vi "EditAxisSpaceCfg_Dialog.vi"(2 "error in":errorcluster, 3 "default save path":path) -> (0 "error out":errorcluster, 1 "Cancelled?":bool)   [LabVIEW 2009]
uses:
  typedefs/AxisSpaceCfg.ctl
  typedefs/AxisCfg.ctl
  globals/AxisSpace.vi
panel:
  in  "Export":bool
  in  "Import":bool
  in  "Cancel Button":bool
  in  "OK Button":bool
  in  "Axis Space":T1
  # "X-Axis\n(Axis 0)"
  # "Y-Axis\n(Axis 1)"
  # "Z-Axis\n(Axis 2)"
  # "Axis Space\n(Axis 3)"
  # "NOTE: \nThis is the \"broadcast axis\". The only value that is used here is the address which is used to broadcast commands to all axes."
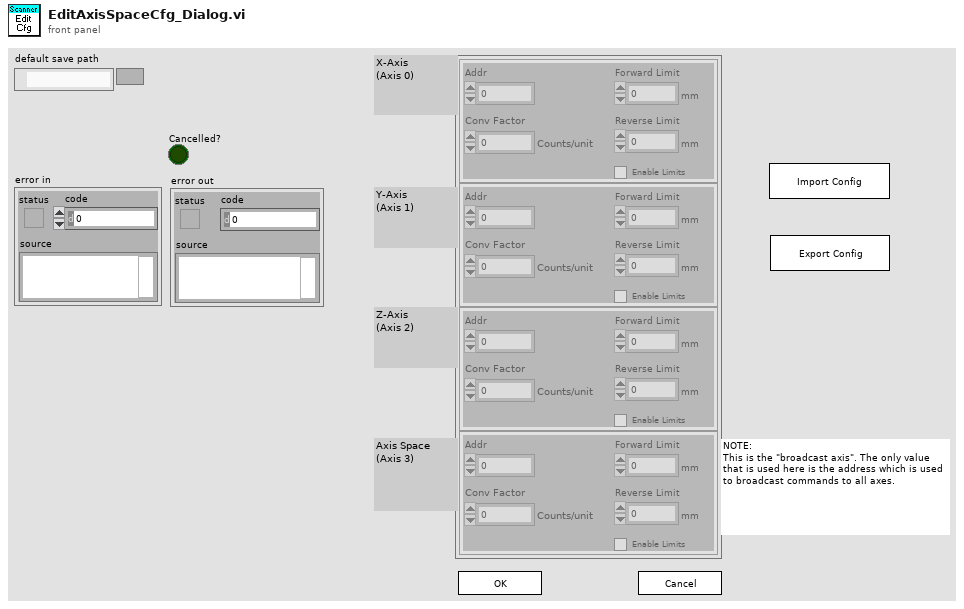
[diagram p1: front panel]
types:
  T1 = typedef "AxisSpaceCfg.ctl" = T2[]
  T2 = typedef "AxisCfg.ctl" = cluster{"Addr":u8, "Conv Factor":dbl, "Forward Limit":dbl, "Reverse Limit":dbl, "Enable Limits":bool}
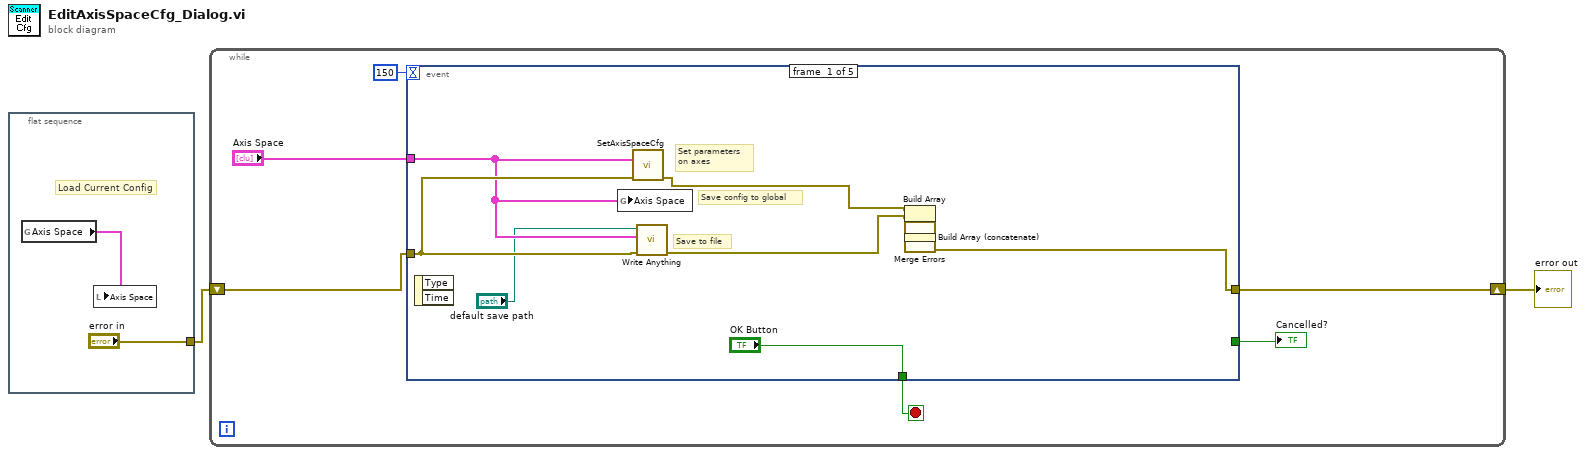
[diagram p0: block diagram]
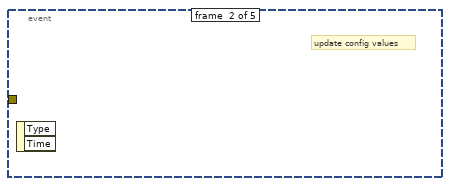
[diagram p2: hidden frame]
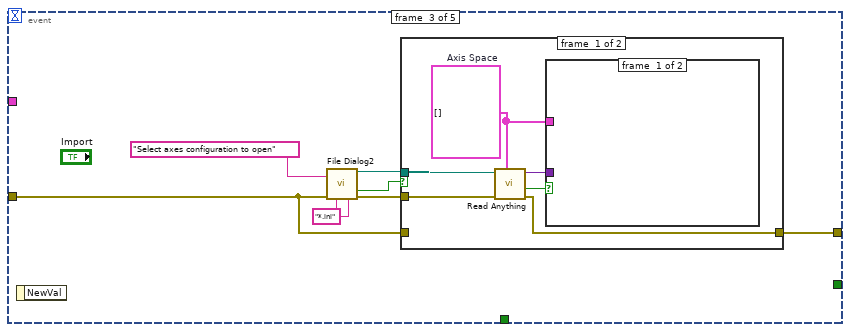
[diagram p3: hidden frame]
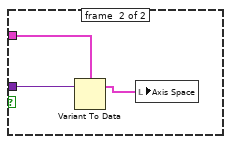
[diagram p4: hidden frame]
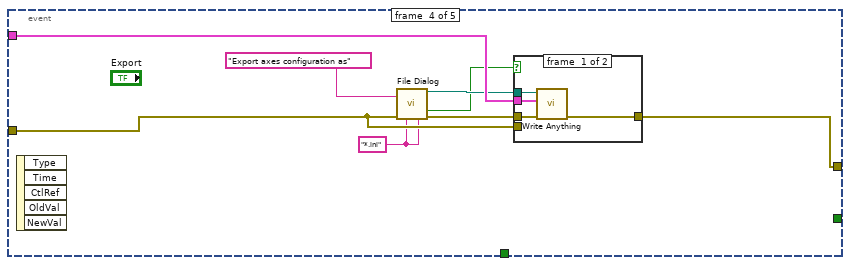
[diagram p6: hidden frame]
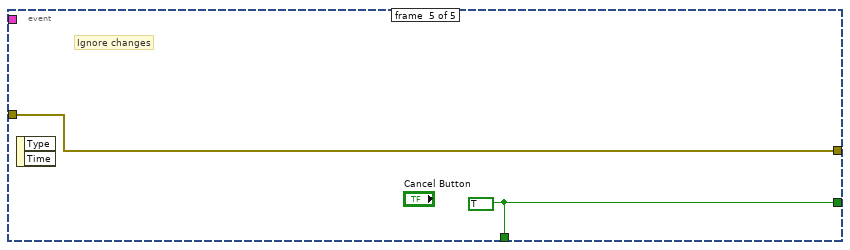
[diagram p8: hidden frame]
diagram:
  n1 = flat-sequence {
    tunnel: ["error in"] -> w2
    frame #0 {
      # "Load Current Config"
      n2 = global read "AxisSpace.vi" "Axis Space"() -> (w3:T1)
      n3 = local write "Axis Space"(w3) -> ()
    }
  }
  n4 = while {
    shift-right: [w7] -> w1
    shift-left: w2 -> [w8]
    stop <- w9 stop-if-true
    n5 = event shown="[4] \"Cancel Button\": Value Change;  Panel Close" {
      selector: _ -> [_ _ _ _ _]
      dyn-events: _ -> [_ _ _ _ _]
      timeout: 150 -> [_ _ _ _ _]
      tunnel: "Axis Space" -> [w12 _ _ w44 _]
      tunnel: ["OK Button" _ _ _ w50] -> w9
      tunnel: [w19 _ w26 w43 w51] -> w7
      tunnel: w8 -> [w18 _ w21 w38 w51]
      tunnel: [_ _ _ _ w50] -> w5
      event #0 {
        # "Save to file"
        # "Set parameters\non axes"
        # "Save config to global"
        n6 = event-data() -> ()  [unwired: 1 in, 2 out]
        n7 = global write "AxisSpace.vi" "Axis Space"(w12) -> ()
        n8 = call "SetAxisSpaceCfg.vi"("Axis Space Config"=w12, "error in (no error)"=w18) -> ("error out"=w15:errorcluster)  [unwired: 13 in]
        n9 = call "Write Anything.vi"("Error In"=w18, "Anything"=w12, "Path (dialog)"="default save path") -> ("Error Out"=w16:errorcluster)  [unwired: 8 in]
        n10 = Build Array(w15, w16) -> (w14:errorcluster[])
        n11 = Build Array (concatenate)(w14) -> (w13:errorcluster[])
        n12 = call <vilib>:"Merge Errors.vi"("error array in"=w13) -> ("error out"=w19:errorcluster)  [unwired: 6 in]
      }
      event #1 {
        # "update config values"
        n13 = event-data() -> ()  [unwired: 1 in, 2 out]
      }
      event #2 {
        w20 = "*.ini" ("pattern (all files)")
        n14 = event-data() -> ()  [unwired: 1 in, 1 out]
        n15 = call "File Dialog2"("prompt"="Select axes configuration to open", "error in"=w21, "pattern (all files)"=w20, "pattern label"=w20) -> ("selected path"=w22:path, "cancelled"=w24:bool, "error out"=w23:errorcluster)  [unwired: 8 in, 1 out]
        n16 = case shown="False" w24 {
          tunnel: w23 -> [w31 _]
          tunnel: w22 -> [w30 _]
          tunnel: [w29 w36] -> w26
          tunnel: w21 -> [_ w36]
          frame #0 {
            w27 = T1 []  # Axis Space
            n17 = call "Read Anything.vi"("Type of Anything"=w27, "Error In"=w31, "Path (dialog)"=w30) -> ("Error Out"=w29:errorcluster, "Found?"=w32:bool, "Anything"=w28:variant)  [unwired: 6 in]
            n18 = case shown="False" w32 {
              tunnel: w28 -> [_ w35]
              tunnel: w27 -> [_ w33]
              frame #0 {
              }
              frame #1 {
                n19 = Variant To Data(Variant=w35, type=w33) -> (data=w34:T1)  [unwired: 1 in, 1 out]
                n20 = local write "Axis Space"(w34) -> ()
              }
            }
          }
          frame #1 {
          }
        }
      }
      event #3 {
        w37 = "*.ini" ("pattern (all files)")
        n21 = event-data() -> ()  [unwired: 1 in, 5 out]
        n22 = call "File Dialog"("prompt"="Export axes configuration as", "error in"=w38, "pattern (all files)"=w37, "pattern label"=w37) -> ("selected path"=w42:path, "cancelled"=w39:bool, "error out"=w41:errorcluster)  [unwired: 8 in, 1 out]
        n23 = case shown="False" w39 {
          tunnel: w42 -> [w48 _]
          tunnel: w44 -> [w45 _]
          tunnel: w41 -> [w47 _]
          tunnel: [w46 w49] -> w43
          tunnel: w38 -> [_ w49]
          frame #0 {
            n24 = call "Write Anything.vi"("Error In"=w47, "Anything"=w45, "Path (dialog)"=w48) -> ("Error Out"=w46:errorcluster)  [unwired: 8 in]
          }
          frame #1 {
          }
        }
      }
      event #4 {
        w50 = TRUE ("OK Button")
        # "Ignore changes"
        n25 = event-data() -> ()  [unwired: 1 in, 2 out]
      }
    }
    "Cancelled?" <- w5
  }
  "error out" <- w1
